vi "IAI Sim.vi"() -> ()   [LabVIEW 2018]
panel:
  out "Alarm Display":string
  in  "Alarm":u16
  out "0207 SON":bool
  out "0206 RES 1":bool
  out "0205 CSTR 1":bool
  out "0204 STP 1":bool
  out "0203 HOME":bool
  out "0202 POS#3":bool
  out "0201 POS#2":bool
  out "0200 POS#1":bool
  in  "0308 PEND1":bool
  in  "0307 HEND1":bool
  in  "0303 MOVE1":bool
  # "OTHER"
  # "Input"
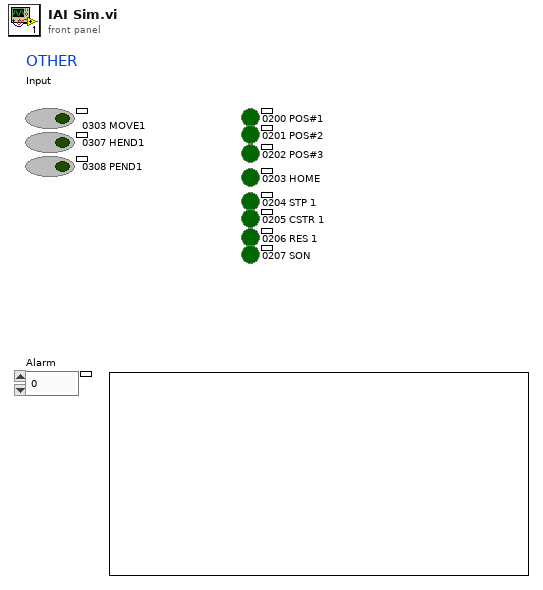
[diagram p1: front panel]
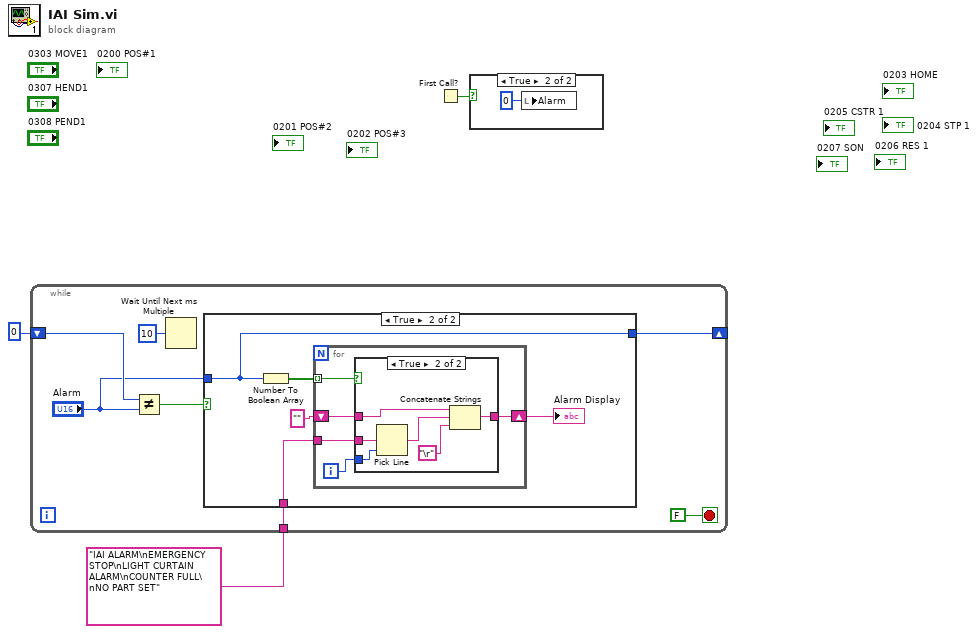
[diagram p0: block diagram]
diagram:
  n1 = while {
    tunnel: "IAI ALARM\nEMERGENCY STOP\nLIGHT CURTAIN ALARM\nCOUNTER FULL\nNO PART SET" -> [w8]
    shift-right: [w5] -> _
    shift-left: u16 0 -> [w7]
    stop <- FALSE stop-if-true
    n2 = Not Equal?(x=w7, y="Alarm") -> (x != y?=w6:bool)
    n3 = Wait Until Next ms Multiple(millisecond multiple=u32 10) -> ()  [unwired: 1 out]
    n4 = case shown="True" w6 {
      tunnel: w8 -> [_ w16]
      tunnel: [w11 w12] -> w5
      tunnel: "Alarm" -> [w11 w12]
      frame False {
      }
      frame True {
        n5 = Number To Boolean Array(number=w12) -> (Boolean array=w15:bool[])
        n6 = for {
          tunnel: w15 -> [w21] mode=indexing
          shift-right: [w18] -> w14
          shift-left: "" -> [w17]
          tunnel: w16 -> [w19]
          i -> [w20]
          n7 = case shown="True" w21 {
            tunnel: w20 -> [_ w28]
            tunnel: w19 -> [_ w27]
            tunnel: w17 -> [w22 w25]
            tunnel: [w22 w26] -> w18
            frame False {
            }
            frame True {
              n8 = Pick Line(multi-line string=w27, line index=w28) -> (output string=w24:string)  [unwired: 1 in]
              n9 = Concatenate Strings(w25, w24, "\r") -> (w26:string)
            }
          }
        }
        "Alarm Display" <- w14
      }
    }
  }
  n10 = First Call?() -> (First Call?: T/F=w2:bool)
  n11 = case shown="True" w2 {
    frame False {
    }
    frame True {
      n12 = local write "Alarm"(u16 0 ("Alarm")) -> ()
    }
  }
